vi "Get settings chain.vi"(8 "error in (no error)":errorcluster, 11 "RSABase in":refnum<class "RSA.lvclass">) -> (0 "error out":errorcluster, 1 "class name":string[](array[string]), 2 "settings":variant[](array[variant]), 3 "RSABase out":refnum<class "RSA.lvclass">)   [LabVIEW 2012, in "RSA.lvclass"]
doc: "Returns an array of variants containing the settings clusters of each class in the inheritance chain (lowest child class first), together with an array of all class names in the inheritance chain.\n\nFor classes without settings cluster, the settings chain contains empty variants."
uses:
  RSA.lvclass
  <vilib>/Distrio/Murmex/Murmex/Murmex.lvclass
  RSA.lvclass/RSA.ctl
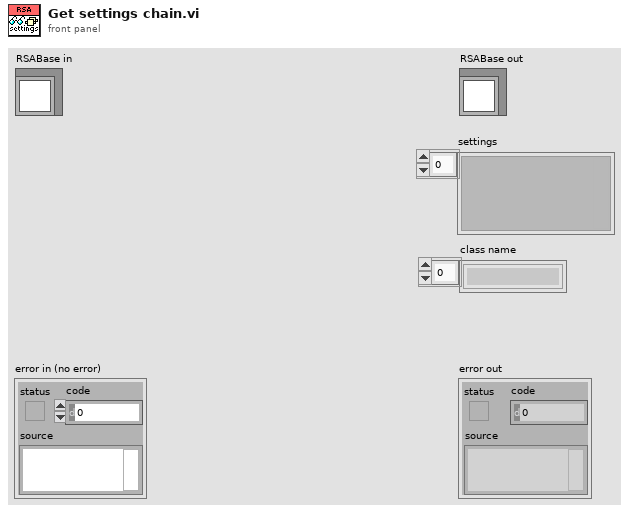
[diagram p1: front panel]
types:
  T1 = typedef "RSA.lvclass/settingscluster.ctl" = cluster{"Search Range percentage":dbl, "Wait time":u32, "stop after":i32, "Iterations untill bleaching compensation":i32, "bunch for bleaching compensation":i32}
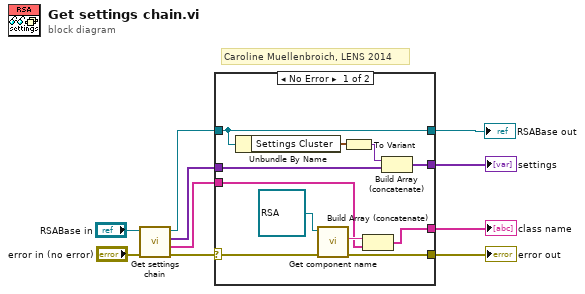
[diagram p0: block diagram]
diagram:
  # "Caroline Muellenbroich, LENS 2014"
  n1 = call-parent "Get settings chain.vi"("error in (no error)"="error in (no error)", "MurmexBase in"="RSABase in") -> ("error out"=w8:errorcluster, "class name"=w5:string[], "settings"=w6:variant[], "MurmexBase out"=w7:refnum<class "RSA.lvclass">)  [unwired: 6 in]
  n2 = case shown="No Error" w8 {
    selector: w8 -> [w16 w25]
    tunnel: w7 -> [w11 w22]
    tunnel: w6 -> [w19 w23]
    tunnel: w5 -> [w14 w24]
    tunnel: [w11 w22] -> w3
    tunnel: [w18 w23] -> w4
    tunnel: [w15 w25] -> w2
    tunnel: [w13 w24] -> w1
    frame No Error {
      n3 = Unbundle By Name(w11) -> ("Settings Cluster"=w21:T1)
      n4 = call <vilib>:"Get component name.vi"("error in (no error)"=w16, "Murmex in"=refnum<class "RSA.lvclass"> refnum ("RSA")) -> ("error out"=w15:errorcluster, "component name"=w17:string)  [unwired: 7 in, 1 out]
      n5 = To Variant(anything=w21) -> (Variant=w20:variant)
      n6 = Build Array (concatenate)(w17, w14) -> (w13:string[])
      n7 = Build Array (concatenate)(w20, w19) -> (w18:variant[])
    }
    frame Error {
    }
  }
  "error out" <- w2
  "RSABase out" <- w3
  "settings" <- w4
  "class name" <- w1
